vi "Under_Body_Wash.vi"(0 "Car_Wash_Data_In":T1) -> (4 "Car_Wash_Data_Out":T1)   [LabVIEW 2021]
doc: "Updates the process of Under body wash in queue"
uses:
  Control/Stage_Data.ctl
  Control/Car_Wash_Indicators.ctl
  Control/Car_Wash_Data.ctl
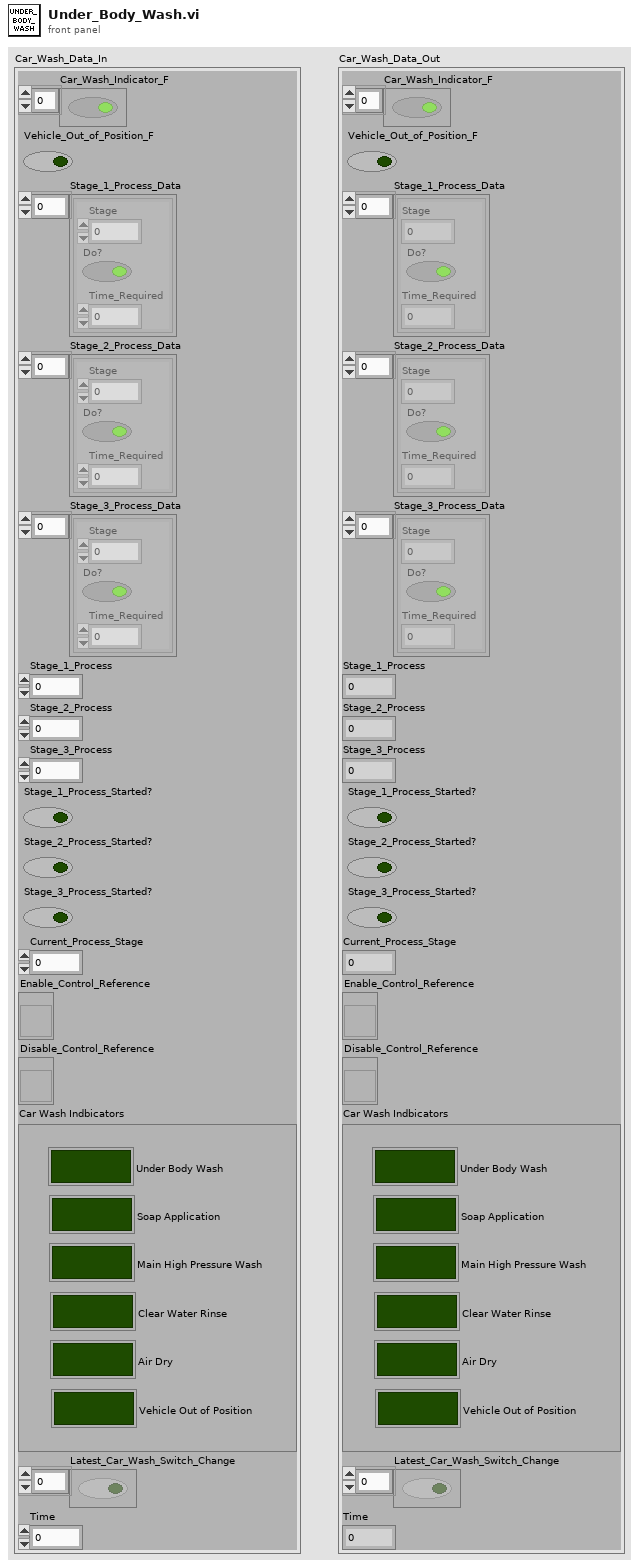
[diagram p1: front panel]
types:
  T1 = typedef "Car_Wash_Data.ctl" = cluster{"Car_Wash_Indicator_F":bool[], "Vehicle_Out_of_Position_F":bool, "Stage_1_Process_Data":T2[], "Stage_2_Process_Data":T2[], "Stage_3_Process_Data":T2[], "Stage_1_Process":i32, "Stage_2_Process":i32, "Stage_3_Process":i32, "Stage_1_Process_Started?":bool, "Stage_2_Process_Started?":bool, "Stage_3_Process_Started?":bool, "Current_Process_Stage":i32, "Enable_Control_Reference":refnum<vi>, "Disable_Control_Reference":refnum<vi>, "Car_Wash_Indicators":T3, "Latest_Car_Wash_Switch_Change":bool[], "Time":dbl}
  T2 = typedef "Stage_Data.ctl" = cluster{"Stage":i32, "Do?":bool, "Time_Required":i32}
  T3 = typedef "Car_Wash_Indicators.ctl" = cluster{"Under_Body_Wash":bool, "Soap_Application":bool, "Main_High_Pressure_Wash":bool, "Clear_Water_Rinse":bool, "Air_Dry":bool, "Vehicle_Out_of_Position":bool}
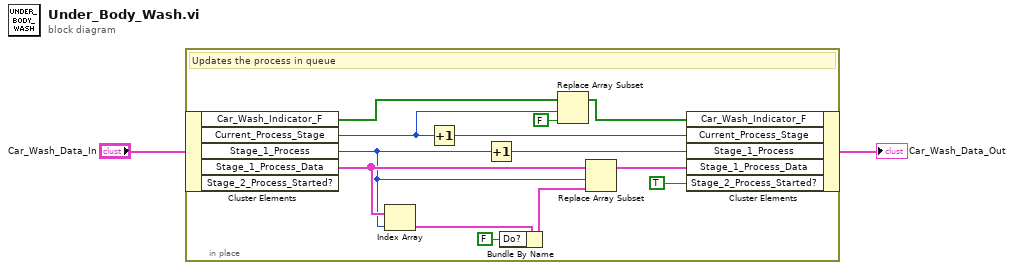
[diagram p0: block diagram]
diagram:
  n1 = in-place "In Place Element Structure" {
    # "Updates the process in queue"
    n2 = in-place-cluster #1("Car_Wash_Data_In") -> ("Car_Wash_Indicator_F"=w9:bool[], "Current_Process_Stage"=w7:i32, "Stage_1_Process"=w5:i32, "Stage_1_Process_Data"=w12:T2[])  [unwired: 1 out]
    n3 = Index Array(array=w12, index=w5) -> (element=w13:T2)
    n4 = Increment(x=w7) -> (x+1=w15:i32)
    n5 = Increment(x=w5) -> (x+1=w10:i32)
    n6 = Bundle By Name(cluster=w13, "Do?"=FALSE) -> (w14:T2)
    n7 = Replace Array Subset(array=w9, new element=FALSE ("new element/subarray"), index=w7) -> (w8:bool[])
    n8 = Replace Array Subset(array=w12, new element=w14, index=w5) -> (w11:T2[])
    n9 = in-place-cluster #1("Car_Wash_Indicator_F"=w8, "Current_Process_Stage"=w15, "Stage_1_Process"=w10, "Stage_1_Process_Data"=w11, "Stage_2_Process_Started?"=TRUE ("Stage_3_Process_Started?")) -> (→"Car_Wash_Data_Out":T1)
  }
